vi "Configuration Keys.vi"(8 "error in":errorcluster, 11 "Electronic Load in":refnum<class "Electronic Load.lvclass">) -> (0 "error out":errorcluster, 2 "Required Keys":string[](array[string]), 3 "Electronic Load out":refnum<class "Electronic Load.lvclass">)   [LabVIEW 2019, in "Electronic Load.lvlib" / "Electronic Load.lvclass"]
doc: "Configuration Keys is a dynamic dispatch VI that reads a full inheritance chain's required key list.\n\nThis means each instrument must override this vi, and call the parent method . The end result is a comprehensive list of required keys that must be present in an instrument's config.ini file to correctly function."
uses:
  Library/Electronic Load.lvclass
  Custom Controls/Configuration Keys.ctl
  builds/Instruments/Instruments.lvlibp/Library/Instruments.lvclass
panel:
  in  "Configuration Keys":T1
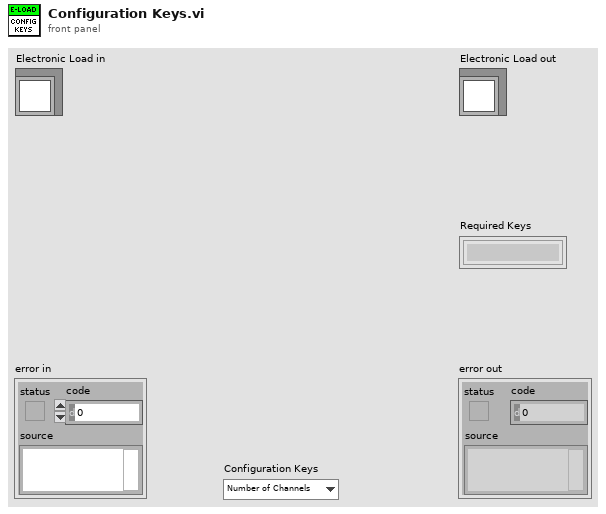
[diagram p1: front panel]
types:
  T1 = typedef "Electronic Load.lvlib/Electronic Load.lvclass/Configuration Keys.ctl" = enum16{"Number of Channels"}
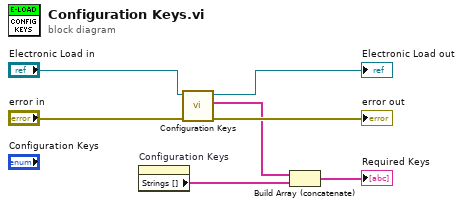
[diagram p0: block diagram]
diagram:
  n1 = property on="Configuration Keys" class="Enum (strict)"() -> ("Strings []"=w3:string[])  [unwired: 2 in, 2 out]
  n2 = call-parent "Configuration Keys.vi"("error in"="error in", "Instruments in"="Electronic Load in") -> ("error out"=→"error out":errorcluster, "Required Keys"=w2:string[], "Instruments out"=→"Electronic Load out":refnum<class "Electronic Load.lvclass">)  [unwired: 7 in]
  n3 = Build Array (concatenate)(w2, w3) -> (→"Required Keys":string[])
